vi "Calculate Process Time.vi"(8 "error in (no error)":errorcluster, 10 "Seconds":dbl, 11 "Model in":refnum<class "Model.lvclass">) -> (0 "error out":errorcluster, 2 "Time":dbl, 3 "Model out":refnum<class "Model.lvclass">)   [LabVIEW 2016, in "Model.lvclass"]
uses:
  Model.lvclass
  Model.lvclass/Model.ctl
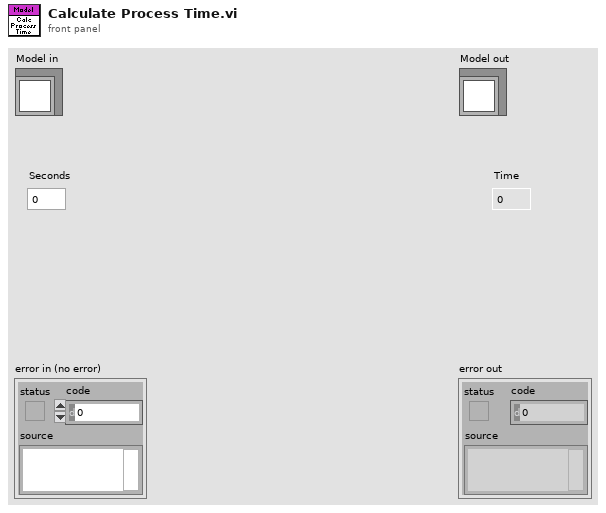
[diagram p1: front panel]
types:
  T1 = typedef "FAMT Typedefs.lvlib/ActuatorData.ctl" = cluster{"Timestamp":dbl, "Axial Force":dbl, "Lateral Force":dbl, "FC1 Force":dbl, "FC2 Force":dbl, "Lateral Push Pressure":dbl, "Lateral Pull Pressure":dbl, "Axial Push Pressure":dbl, "Axial Pull Pressure":dbl}
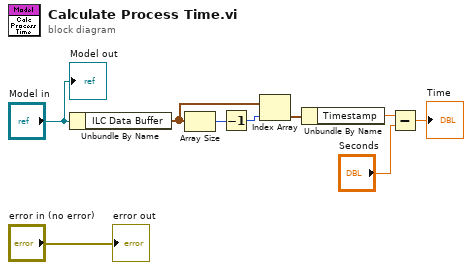
[diagram p0: block diagram]
diagram:
  n1 = Unbundle By Name("Model in") -> ("ILC Data Buffer"=w4:T1[])
  n2 = Array Size(array=w4) -> (size(s)=w9:i32)
  n3 = Decrement(x=w9) -> (x-1=w8:i32)
  n4 = Index Array(array=w4, index=w8) -> (element=w7:T1)
  n5 = Unbundle By Name(w7) -> ("Timestamp"=w6:dbl)
  n6 = Subtract(x=w6, y="Seconds") -> (x-y=→"Time":dbl)
  "error out" <- "error in (no error)"
  "Model out" <- "Model in"
